vi "cRIO Read Module Model.vi"(8 "error in (no error)":errorcluster, 11 "Refnum in":T1) -> (0 "error out":errorcluster, 2 "Module Model":string, 3 "Refnum out":T1)   [LabVIEW 2017, in "cRIODetectHW.lvlib"]
uses:
  <vilib>/addons/cRIODetectHW/cRIODetectHW.lvlib
  <vilib>/addons/cRIODetectHW/control/FPGARef.ctl
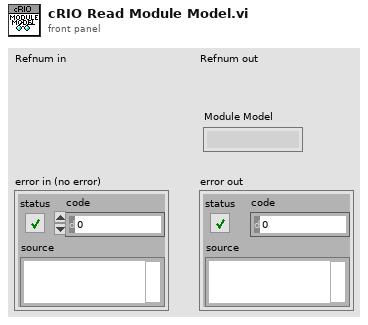
[diagram p1: front panel]
types:
  T1 = typedef "cRIODetectHW.lvlib/FPGARef.ctl" = refnum<k20>
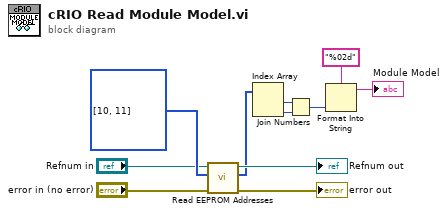
[diagram p0: block diagram]
diagram:
  n1 = call <vilib>:"Read EEPROM Addresses.vi"("error in (no error)"="error in (no error)", "Addresses"=u16[] [10, 11], "Refnum in"="Refnum in") -> ("error out"=→"error out":errorcluster, "Data"=w4:u8[], "Refnum out"=→"Refnum out":T1)  [unwired: 6 in]
  n2 = Index Array(array=w4) -> (element #1=w2:u8, element #2=w3:u8)  [unwired: 2 in]
  n3 = Join Numbers(hi=w2, lo=w3) -> ((hi.lo)=w1:u16)
  n4 = Format Into String(format string="%02d", w1) -> (resulting string=→"Module Model":string)  [unwired: 2 in, 1 out]
